vi "Configure Parameter SQU.vi"(7 "PARAM":enum16{"POL", "GRO"}(ring), 8 "error in (no error)":errorcluster, 9 "STAT@POL":enum16{"POS", "NEG", "SYMM"}(ring), 10 "STAT@GRO":enum16{"ON", "OFF"}(ring), 11 "VISA resource name":refnum<visa-resource-name>) -> (0 "error out":errorcluster, 3 "VISA resource name out":refnum<visa-resource-name>)   [LabVIEW 2018, in "Fluke 9500B.lvlib"]
uses:
  <instrlib>/Fluke 9500B/Fluke 9500B.lvlib
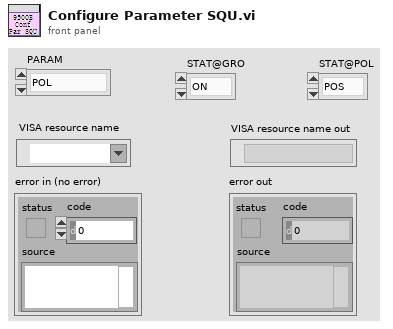
[diagram p1: front panel]
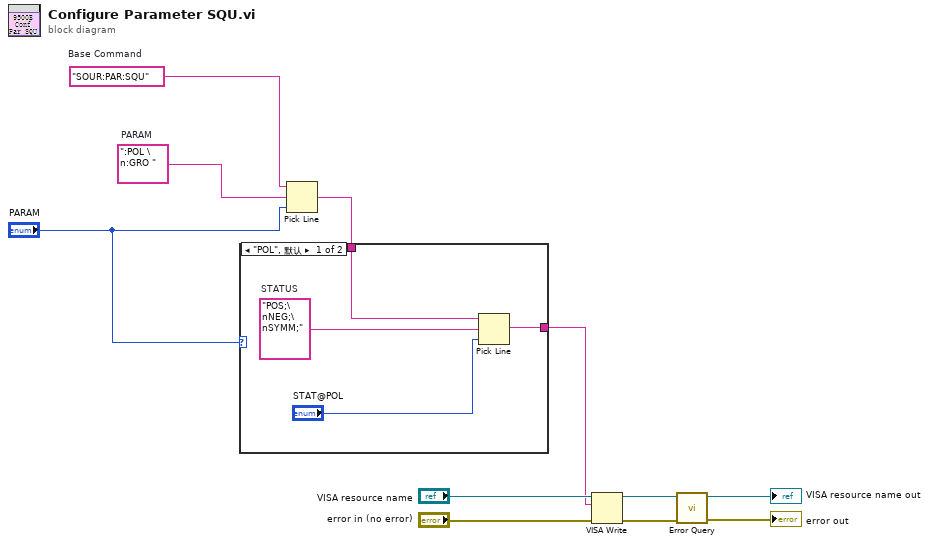
[diagram p0: block diagram]
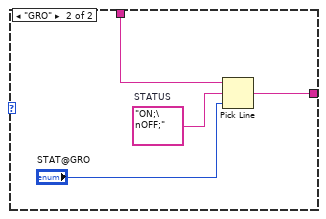
[diagram p2: hidden frame]
diagram:
  w8 = ":POL \n:GRO "  # PARAM
  w9 = "SOUR:PAR:SQU"  # Base Command
  n1 = Pick Line(string ("")=w9, multi-line string=w8, line index="PARAM") -> (output string=w7:string)
  n2 = case shown="\"POL\", 默认" "PARAM" {
    tunnel: w7 -> [w13 w19]
    tunnel: [w12 w18] -> w6
    frame "POL", Default {
      w15 = "POS;\nNEG;\nSYMM;"  # STATUS
      n3 = Pick Line(string ("")=w13, multi-line string=w15, line index="STAT@POL") -> (output string=w12:string)
    }
    frame "GRO" {
      w17 = "ON;\nOFF;"  # STATUS
      n4 = Pick Line(string ("")=w19, multi-line string=w17, line index="STAT@GRO") -> (output string=w18:string)
    }
  }
  n5 = VISA Write(VISA resource name="VISA resource name", write buffer=w6, error in (no error)="error in (no error)") -> (VISA resource name out=w4:refnum<visa-resource-name>, error out=w3:errorcluster)  [unwired: 1 out]
  n6 = call <instrlib>:"Error Query.vi"("error in (no error)"=w3, "VISA resource name"=w4) -> ("error out"=→"error out":errorcluster, "VISA resource name out"=→"VISA resource name out":refnum<visa-resource-name>)  [unwired: 6 in, 2 out]
